vi "write single coil.vi"(8 "error in (no error)":errorcluster, 10 "value":bool, 11 "address":u16) -> (0 "error out":errorcluster)   [LabVIEW 2016, in "环境动力监测库.lvlib" / "浮标电源管理.lvlib"]
uses:
  <vilib>/Plasmionique/MB Master/MB Master.lvlib
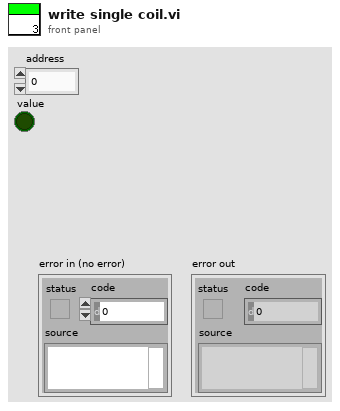
[diagram p1: front panel]
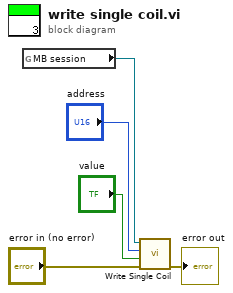
[diagram p0: block diagram]
diagram:
  n1 = global read "通讯全局变量.vi" "MB session"() -> (w5:refnum<class "MB_Master.lvclass">)
  n2 = call <vilib>:"Write Single Coil.vi"("error in (no error)"="error in (no error)", "value"="value", "address"="address", "MB session in"=w5) -> ("error out"=→"error out":errorcluster)  [unwired: 6 in, 1 out]
